vi "wrapcutlifetime.vi"(0 "lineshift":i32) -> (1 "pt3img":u16[][](array[numeric]), 2 "lifetimes":sgl[][](array[numeric]) format="%.2f", 3 "okay":bool, 4 "# of frames":i32)   [LabVIEW 2015]
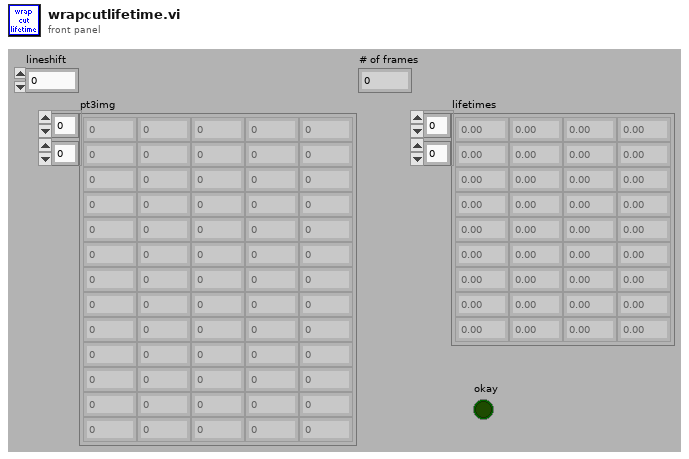
[diagram p1: front panel]
types:
  T1 = typedef "LVRectTypeDef.ctl" = cluster{"Left":i16, "Top":i16, "Right":i16, "Bottom":i16}
  T2 = cluster{"Xpixels":i32, "Vxminref":dbl, "Vxmaxref":dbl, "P":dbl, "Ypixels":i32, "Vyminref":dbl, "Vymaxref":dbl, "srate":sgl, "sAOxy":i32, "timeout":dbl, "type":string, "date":string, "time":string, "Colormap":u16, "Drawing Mode":u16, "Scanning Mode":u16, "square pixels":bool, "square matrix":bool, "Xpixels Img":i32, "Vx-min Img":dbl, "VX-max Img":dbl, "Ypixels Img":i32, "Vy-min Img":dbl, "Vy-max Img ":dbl, "Angle Img":dbl, "autoshutter":bool, "finite":bool, "cont":bool, "wavdet":bool, "measpoints":i32, "avpp":i32, "bufferAO":i32, "bufferAI":i32, "starttick":u32, "waveform":path, "Vx-ref":dbl, "Vy-ref":dbl, "refreshrate":dbl, "refreshbuffer":i32, "tt_cycles":i32, "motorref":refnum<k7>, "mirrorswitch":refnum<k7>, "sample mode":i32, "maxbufferAI":i32, "srateAODO":sgl, "bin":sgl, "Pel":sgl, "Angle draw":dbl, "srate Img":sgl, "ROIimg_plotbounds":T1, "auto OD":bool, "ODfilt":u16, "aAI":i32[], "aCI":i32[], "aAO":u32[], "aDO":u32[], "refwfsize":dbl, "Lifetime":bool, "Vz-Img":dbl, "Vz-ref":dbl, "Vz-reset":dbl, "AIoverride":bool}
  T3 = cluster{"initialized":bool, "devidx":i32, "Ch0 Level":i32, "Ch0 ZeroX":i32, "Ch1 Level":i32, "Ch1 ZeroX":i32, "sync rate":i32, "resolution":i32, "acq time":i32, "acq rate":i32, "# bins":u32, "Bin size":enum16{"1", "2", "4", "8", "16", "32", "64", "128"}, "min photons":u32, "truncate":u32}
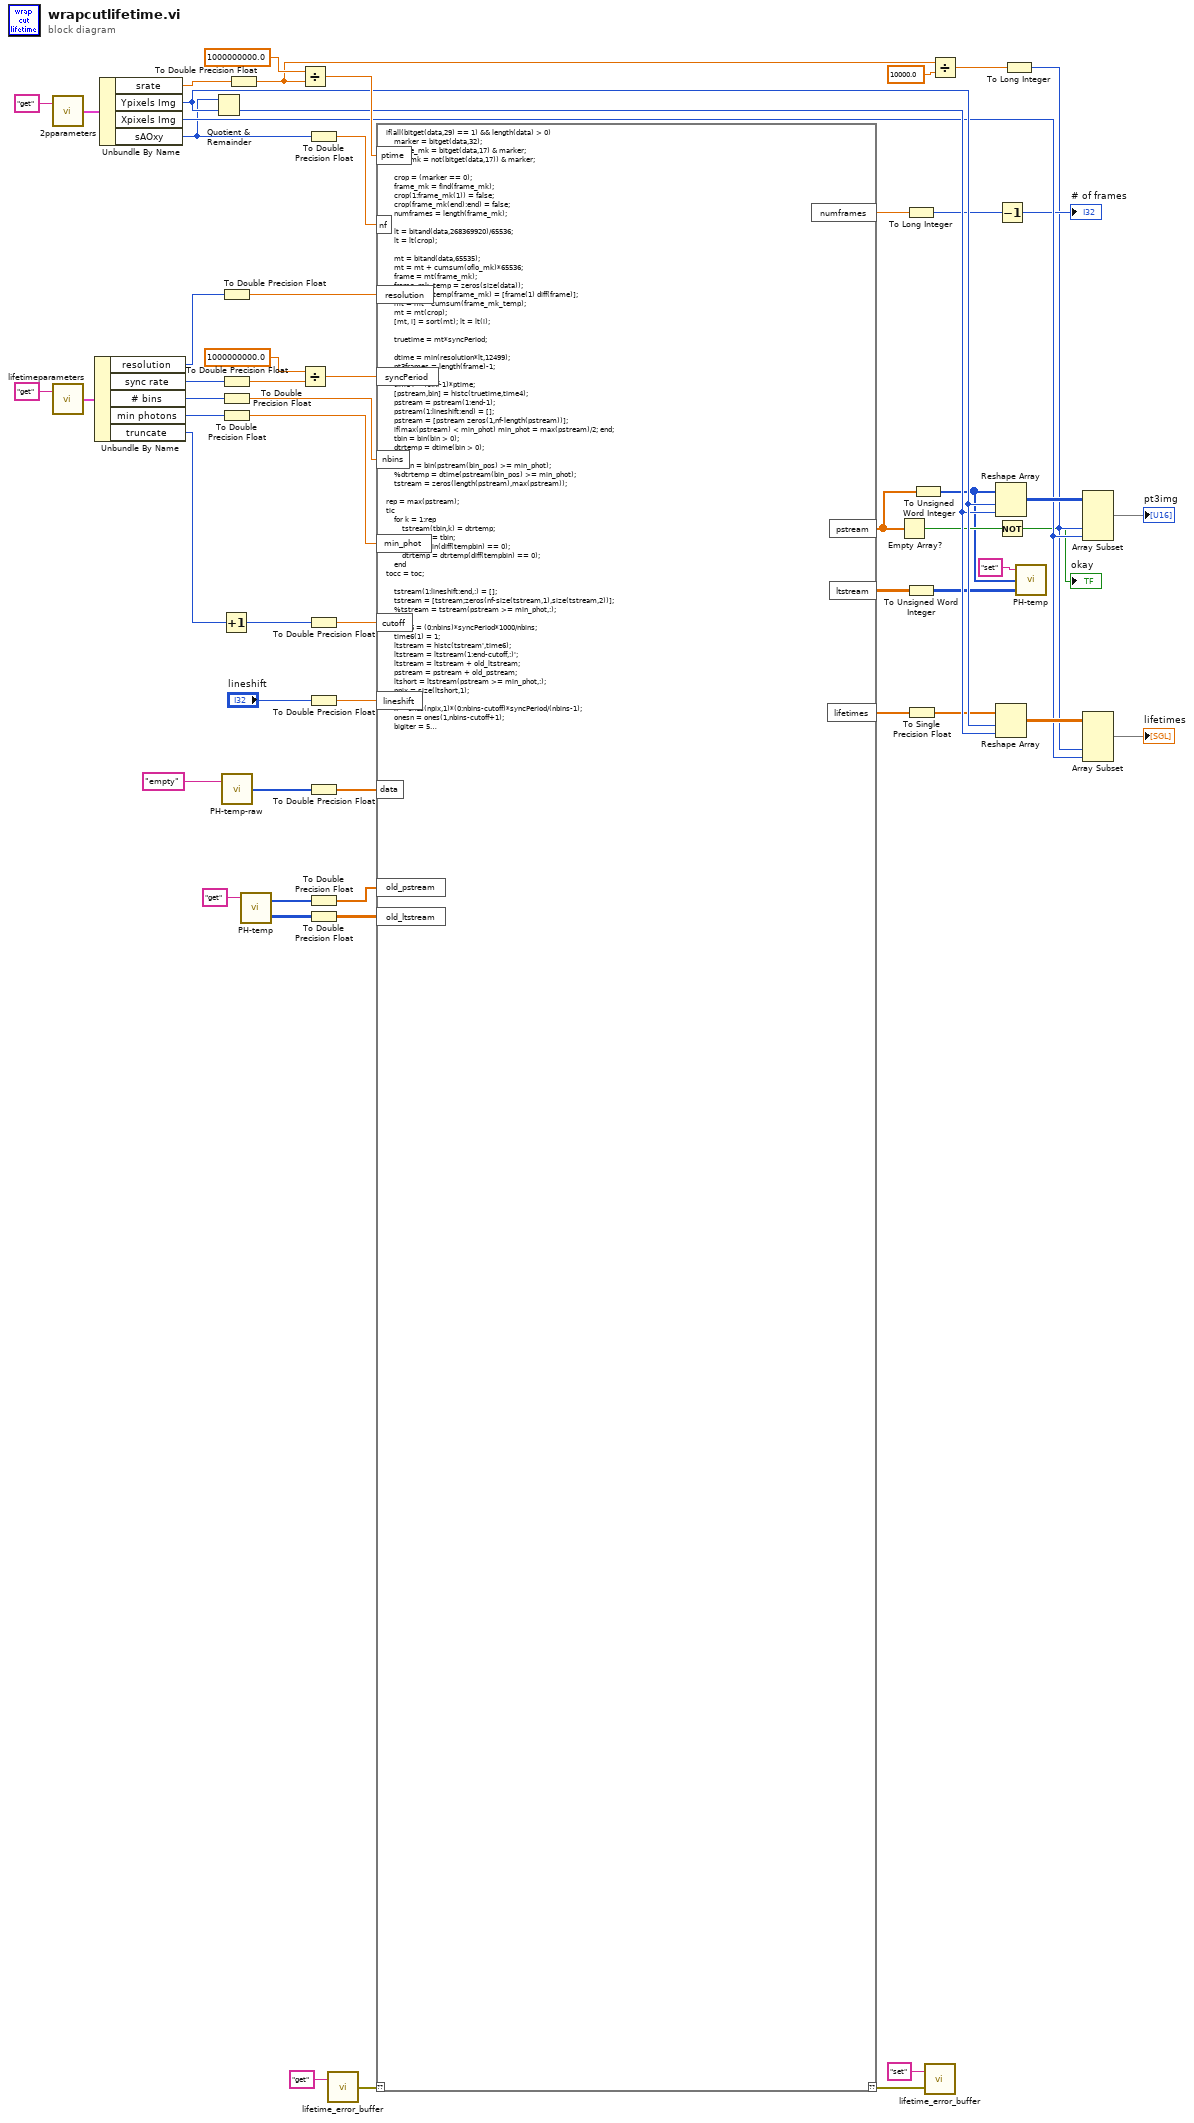
[diagram p0: block diagram]
diagram:
  n1 = call "2pparameters.vi"("command"="get") -> ("params out"=w58:T2)  [unwired: 1 in]
  n2 = call "lifetimeparameters.vi"("command"="get") -> ("Params out"=w49:T3)  [unwired: 1 in]
  n3 = Unbundle By Name(w49) -> ("resolution"=w46:i32, "sync rate"=w45:i32, "# bins"=w33:u32, "min photons"=w9:u32, "truncate"=w3:u32)
  n4 = Unbundle By Name(w58) -> ("srate"=w47:sgl, "Ypixels Img"=w39:i32, "Xpixels Img"=w35:i32, "sAOxy"=w29:i32)
  n5 = Quotient & Remainder(x=w29, y=w39) -> (floor(x/y)=w37:i32)  [unwired: 1 out]
  n6 = Increment(x=w3) -> (x+1=w2:u32)
  n7 = To Double Precision Float(number=w46) -> (double precision float=w56:dbl)
  n8 = To Double Precision Float(number=w45) -> (double precision float=w55:dbl)
  n9 = To Double Precision Float(number=w33) -> (double precision float=w32:dbl)
  n10 = To Double Precision Float(number=w9) -> (double precision float=w19:dbl)
  n11 = call "PH-temp-raw.vi"("command"="empty") -> ("array out"=w44:u32[])  [unwired: 1 in]
  n12 = To Double Precision Float(number=w47) -> (double precision float=w27:dbl)
  n13 = call "PH-temp.vi"("String"="get") -> ("ltstream out"=w8:u16[][], "pstream out"=w12:u16[])  [unwired: 2 in]
  n14 = Divide(x=1000000000.0, y=w27) -> (x/y=w53:dbl)
  n15 = Divide(x=1000000000.0, y=w55) -> (x/y=w50:dbl)
  n16 = To Double Precision Float(number=w29) -> (double precision float=w43:dbl)
  n17 = To Double Precision Float(number=w2) -> (double precision float=w4:dbl)
  n18 = To Double Precision Float(number="lineshift") -> (double precision float=w30:dbl)
  n19 = To Double Precision Float(number=w44) -> (double precision float=w54:dbl[])
  n20 = To Double Precision Float(number=w12) -> (double precision float=w11:dbl[])
  n21 = To Double Precision Float(number=w8) -> (double precision float=w7:dbl[][])
  n22 = call "lifetime_error_buffer.vi"("command"="get") -> ("error out"=w20:errorcluster)  [unwired: 1 in]
  n23 = script code="if(all(bitget(data,29) == 1) && length(data) > 0)\n    marker = bitget(data,32);\n    frame_mk = bitget(data,17) & marker;\n    oflo_mk = not(bitget(data,17)) & marker;\n\n    crop = (marker == 0);\n    frame_mk = find(frame_mk);\n    crop(1:frame_mk(1)) = false;\n    crop(frame_mk(end):end) = false;\n    numframes = length(frame_mk);\n\n    lt = bitand(data,268369920)/65536;\n    lt = lt(crop);\n\n    mt = bitand(data,65535);\n    mt = mt + cumsum(oflo_mk)*65536;\n    frame = mt(frame_mk);\n    frame_mk_temp = zeros(size(data));\n    frame_mk_temp(frame_mk) = [frame(1) diff(frame)];\n    mt = mt - cumsum(frame_mk_temp);\n    mt = mt(crop);\n    [mt, i] = sort(mt); lt = lt(i);\n\n    truetime = mt*syncPeriod;\n\n    dtime = min(resolution*lt,12499);\n    pt3frames = length(frame)-1;\n\n    time4 = (0:nf-1)*ptime;\n    [pstream,bin] = histc(truetime,time4);\n    pstream = pstream(1:end-1);\n    pstream(1:lineshift:end) = [];\n    pstream = [pstream zeros(1,nf-length(pstream))];\n    if(max(pstream) < min_phot) min_phot = max(pstream)/2; end;\n    tbin = bin(bin > 0);\n    dtrtemp = dtime(bin > 0);\n\n    %tbin = bin(pstream(bin_pos) >= min_phot);\n    %dtrtemp = dtime(pstream(bin_pos) >= min_phot);\n    tstream = zeros(length(pstream),max(pstream));\n\nrep = max(pstream);\ntic\n    for k = 1:rep\n        tstream(tbin,k) = dtrtemp;\n        tempbin = tbin;\n        tbin = tbin(diff(tempbin) == 0);\n        dtrtemp = dtrtemp(diff(tempbin) == 0);\n    end\ntocc = toc;\n\n    tstream(1:lineshift:end,:) = [];\n    tstream = [tstream;zeros(nf-size(tstream,1),size(tstream,2))];\n    %tstream = tstream(pstream >= min_phot,:);\n\n    time6 = (0:nbins)*syncPeriod*1000/nbins;\n    time6(1) = 1;\n    ltstream = histc(tstream',time6);\n    ltstream = ltstream(1:end-cutoff,:)';\n    ltstream = ltstream + old_ltstream;\n    pstream = pstream + old_pstream;\n    ltshort = ltstream(pstream >= min_phot,:);\n    npix = size(ltshort,1);\n\n    x = ones(npix,1)*(0:nbins-cutoff)*syncPeriod/(nbins-1);\n    onesn = ones(1,nbins-cutoff+1);\n    bigiter = 50;\n    smalliter = 1;\n    rp = .8;\n\n    a = [ltshort(:,1) ltshort(:,1)*1.5];\n    b1= -abs(log(ltshort(:,2)./ltshort(:,1))./x(:,2));\n    b1(isnan(b1)) = 0; % quick fix for NaN problem\n    b1(isinf(b1)) = 0;\n    b1(b1 == 0) = -.25; % note that this affects the above two cases\n    b = [b1 b1*1.5];\n    c = [zeros(npix,1) 15*ones(npix,1)];\n    fold = zeros(npix,1);\n\n    for i = 1:bigiter\n\n        if max(abs(a(:,1)-a(:,2)),[],1) > 1\n            f1 = a(:,1)*onesn.*exp(b(:,1)*onesn.*x)+c(:,1)*onesn;\n            f2 = a(:,2)*onesn.*exp(b(:,1)*onesn.*x)+c(:,1)*onesn;\n            fv1 = f1-ltshort-ltshort.*log(f1)+ltshort.*log(ltshort);\n            fv1(isnan(fv1)) = f1(isnan(fv1));\n            fv2 = f2-ltshort-ltshort.*log(f2)+ltshort.*log(ltshort);\n            fv2(isnan(fv2)) = f2(isnan(fv2));\n            fv = [sum(fv1,2) sum(fv2,2)];\n            [~,j] = sort(fv,2); \n            a = [(2-j(:,1)).*a(:,1)+(j(:,1)-1).*a(:,2) (2+3*rp-(1+2*rp)*j(:,1)).*a(:,1)+((1+2*rp)*j(:,1)-1-3*rp).*a(:,2)];\n        end\n\n        if max(abs(b(:,1)-b(:,2)),[],1) > .01\n            f1 = a(:,1)*onesn.*exp(b(:,1)*onesn.*x)+c(:,1)*onesn;\n            f2 = a(:,1)*onesn.*exp(b(:,2)*onesn.*x)+c(:,1)*onesn;\n            fv1 = f1-ltshort-ltshort.*log(f1)+ltshort.*log(ltshort);\n            fv1(isnan(fv1)) = f1(isnan(fv1));\n            fv2 = f2-ltshort-ltshort.*log(f2)+ltshort.*log(ltshort);\n            fv2(isnan(fv2)) = f2(isnan(fv2));\n            fv = [sum(fv1,2) sum(fv2,2)];\n            [~,j] = sort(fv,2);\n            b = -abs([(2-j(:,1)).*b(:,1)+(j(:,1)-1).*b(:,2) (2+3*rp-(1+2*rp)*j(:,1)).*b(:,1)+((1+2*rp)*j(:,1)-1-3*rp).*b(:,2)]);\n        end\n\n        if max(abs(c(:,1)-c(:,2)),[],1) > 1\n            f1 = a(:,1)*onesn.*exp(b(:,1)*onesn.*x)+c(:,1)*onesn;\n            f2 = a(:,1)*onesn.*exp(b(:,1)*onesn.*x)+c(:,2)*onesn;\n            fv1 = f1-ltshort-ltshort.*log(f1)+ltshort.*log(ltshort);\n            fv1(isnan(fv1)) = f1(isnan(fv1));\n            fv2 = f2-ltshort-ltshort.*log(f2)+ltshort.*log(ltshort);\n            fv2(isnan(fv2)) = f2(isnan(fv2));\n            fv = [sum(fv1,2) sum(fv2,2)];\n            [~,j] = sort(fv,2); \n            c = [(2-j(:,1)).*c(:,1)+(j(:,1)-1).*c(:,2) (2+3*rp-(1+2*rp)*j(:,1)).*c(:,1)+((1+2*rp)*j(:,1)-1-3*rp).*c(:,2)];\n        end\n\n        if max(abs(fv(:,1)-fold),[],1) <= .01\n            break\n        end\n\n        fold = fv(:,1);\n\n    end\n\n    lttrunc = -syncPeriod./(b(:,1)'*nbins);\n    lifetimes = zeros(size(pstream));\n    lifetimes(pstream >= min_phot) = lttrunc;\nend;"("??"=w20, "syncPeriod"=w50, "resolution"=w56, "ptime"=w53, "nf"=w43, "data"=w54, "nbins"=w32, "lineshift"=w30, "cutoff"=w4, "min_phot"=w19, "old_pstream"=w11, "old_ltstream"=w7) -> ("??"=w1:errorcluster, "pstream"=w17:dbl[], "numframes"=w36:dbl, "lifetimes"=w22:dbl[], "ltstream"=w10:dbl[][])
  n24 = Empty Array?(array=w17) -> (empty?=w16:bool)
  n25 = To Long Integer(number=w36) -> (32bit integer=w18:i32)
  n26 = To Unsigned Word Integer(number=w10) -> (unsigned 16bit integer=w6:u16[][])
  n27 = To Single Precision Float(number=w22) -> (single precision float=w23:sgl[])
  n28 = To Unsigned Word Integer(number=w17) -> (unsigned 16bit integer=w5:u16[])
  n29 = call "lifetime_error_buffer.vi"("error in"=w1, "command"="set") -> ()  [unwired: 1 out]
  n30 = Divide(x=w27, y=10000.0) -> (x/y=w26:dbl)
  n31 = Reshape Array(w5, w39, w37) -> (w42:u16[][])
  n32 = Reshape Array(w23, w39, w37) -> (w40:sgl[][])
  n33 = Decrement(x=w18) -> (x-1=→"# of frames":i32)
  n34 = Not(x=w16) -> (.not. x?=→"okay":bool)
  n35 = To Long Integer(number=w26) -> (32bit integer=w25:i32)
  n36 = call "PH-temp.vi"("ltstream in"=w6, "pstream in"=w5, "String"="set") -> ()  [unwired: 2 out]
  n37 = Array Subset(array=w42, index (col)=w25, length (col)=w35) -> (→"pt3img":u16[][])  [unwired: 2 in]
  n38 = Array Subset(array=w40, index (col)=w25, length (col)=w35) -> (→"lifetimes":sgl[][])  [unwired: 2 in]
